vi "浮动通知3.vi"(10 "通知时间(S)":dbl=3.0, 11 "通知内容":string) -> ()   [LabVIEW 2020]
uses:
  Global_Variable/Global.vi
panel:
  in  "背景颜色":u32(colorbox)
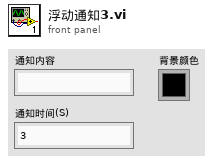
[diagram p1: front panel]
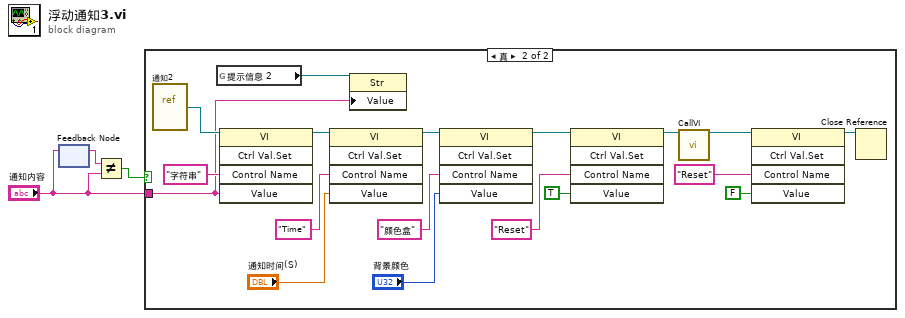
[diagram p0: block diagram]
diagram:
  n1 = feedback-in #1("通知内容") -> ()
  n2 = feedback #1() -> (w2:string)  [unwired: 1 in]
  n3 = Not Equal?(x=w2, y="通知内容") -> (x != y?=w3:bool)
  n4 = case shown="真" w3 {
    tunnel: "通知内容" -> [_ w4]
    frame False {
    }
    frame True {
      n5 = vi-ref "通知2.vi"() -> (w7:refnum<vi>)
      n6 = global read "Global.vi" "提示信息 2"() -> (w5:refnum<vi>)
      n7 = invoke class="VI" method="Ctrl Val.Set"(reference=w7, "Control Name"="字符串" ("控件名"), "Value"=w4) -> (reference out=w6:refnum<vi>)  [unwired: 2 in, 4 out]
      n8 = invoke class="VI" method="Ctrl Val.Set"(reference=w6, "Control Name"="Time" ("控件名"), "Value"="通知时间(S)") -> (reference out=w11:refnum<vi>)  [unwired: 2 in, 4 out]
      n9 = property class="Str"(reference=w5, "Value"=w4) -> ()  [unwired: 1 in, 2 out]
      n10 = invoke class="VI" method="Ctrl Val.Set"(reference=w11, "Control Name"="颜色盒" ("控件名"), "Value"="背景颜色") -> (reference out=w10:refnum<vi>)  [unwired: 2 in, 4 out]
      n11 = invoke class="VI" method="Ctrl Val.Set"(reference=w10, "Control Name"="Reset" ("控件名"), "Value"=TRUE) -> (reference out=w13:refnum<vi>)  [unwired: 2 in, 4 out]
      n12 = call "CallVI.vi"("VI引用"=w13) -> ("VI引用输出"=w12:refnum<vi>)  [unwired: 12 in, 2 out]
      n13 = invoke class="VI" method="Ctrl Val.Set"(reference=w12, "Control Name"="Reset" ("控件名"), "Value"=FALSE) -> (reference out=w14:refnum<vi>)  [unwired: 2 in, 4 out]
      n14 = Close Reference(reference=w14) -> ()  [unwired: 1 in, 1 out]
    }
  }
